vi "lasercontrols.vi"() -> ()   [LabVIEW 2013]
panel:
  in  "637":bool
  in  "488":bool
  in  "stop":bool
  in  "532":bool
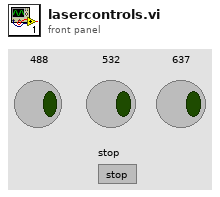
[diagram p1: front panel]
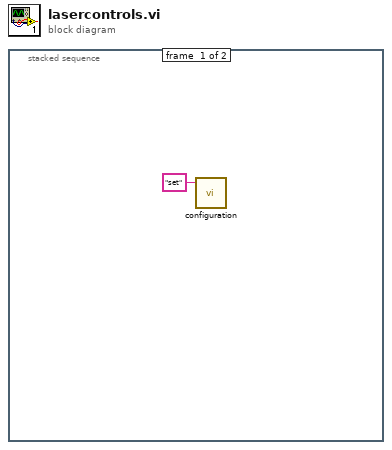
[diagram p0: block diagram]
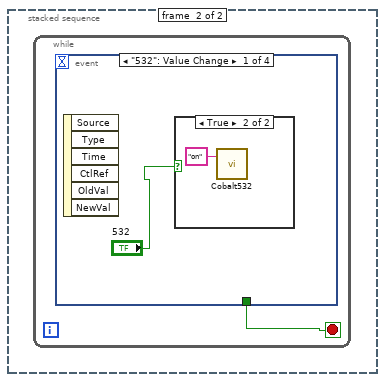
[diagram p2: hidden frame]
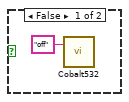
[diagram p3: hidden frame]
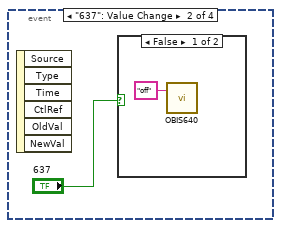
[diagram p4: hidden frame]
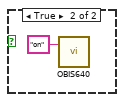
[diagram p5: hidden frame]
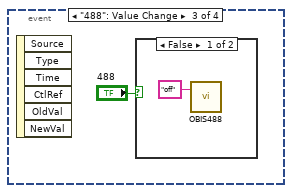
[diagram p6: hidden frame]
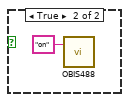
[diagram p7: hidden frame]
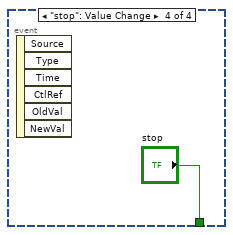
[diagram p8: hidden frame]
diagram:
  n1 = stacked-sequence {
    frame #0 {
      n2 = call "configuration.vi"("command"="set") -> ()  [unwired: 2 in, 2 out]
    }
    frame #1 {
      n3 = while {
        stop <- w2 stop-if-true
        n4 = event shown="[0] \"532\": Value Change" {
          selector: _ -> [_ _ _ _]
          dyn-events: _ -> [_ _ _ _]
          timeout: _ -> [_ _ _ _]
          tunnel: [_ _ _ "stop"] -> w2
          event "532": Value Change {
            n5 = event-data() -> ()  [unwired: 1 in, 6 out]
            n6 = case shown="True" "532" {
              frame False {
                n7 = call "Cobalt532.vi"("command"="off") -> ()  [unwired: 1 in, 1 out]
              }
              frame True {
                n8 = call "Cobalt532.vi"("command"="on") -> ()  [unwired: 1 in, 1 out]
              }
            }
          }
          event "637": Value Change {
            n9 = event-data() -> ()  [unwired: 1 in, 6 out]
            n10 = case shown="False" "637" {
              frame False {
                n11 = call "OBIS640.vi"("command"="off") -> ()  [unwired: 1 in, 1 out]
              }
              frame True {
                n12 = call "OBIS640.vi"("command"="on") -> ()  [unwired: 1 in, 1 out]
              }
            }
          }
          event "488": Value Change {
            n13 = event-data() -> ()  [unwired: 1 in, 6 out]
            n14 = case shown="False" "488" {
              frame False {
                n15 = call "OBIS488.vi"("command"="off") -> ()  [unwired: 1 in, 1 out]
              }
              frame True {
                n16 = call "OBIS488.vi"("command"="on") -> ()  [unwired: 1 in, 1 out]
              }
            }
          }
          event "stop": Value Change {
            n17 = event-data() -> ()  [unwired: 1 in, 6 out]
          }
        }
      }
    }
  }
